vi "解析分辨率.vi"(10 "分辨率":string) -> (1 "number 2":i32, 2 "number":i32)   [LabVIEW 2016]
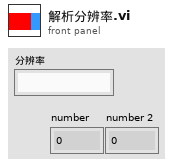
[diagram p1: front panel]
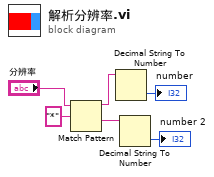
[diagram p0: block diagram]
diagram:
  n1 = Match Pattern(string="分辨率", regular expression="*") -> (before substring=w6:string, after substring=w5:string)  [unwired: 1 in, 2 out]
  n2 = Decimal String To Number(string=w6) -> (number=→"number":i32)  [unwired: 2 in, 1 out]
  n3 = Decimal String To Number(string=w5) -> (number=→"number 2":i32)  [unwired: 2 in, 1 out]
